vi "Set DBC Communication.vi"(8 "error in":errorcluster, 10 "DBC Communication.lvclass":refnum<class "DBC Communication.lvclass">, 11 "HSU MCU V2 in":refnum<class "HSU MCU V2.lvclass">) -> (0 "error out":errorcluster, 3 "HSU MCU V2 out":refnum<class "HSU MCU V2.lvclass">)   [LabVIEW 2024, in "HSU MCU V2.lvclass"]
uses:
  HSU MCU V2.lvclass
  DBCCommunication/DBC Communication.lvclass
  HSU MCU V2.lvclass/HSU MCU V2.ctl
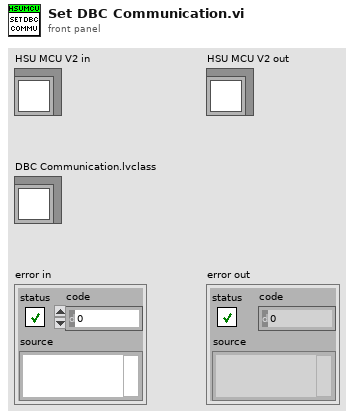
[diagram p1: front panel]
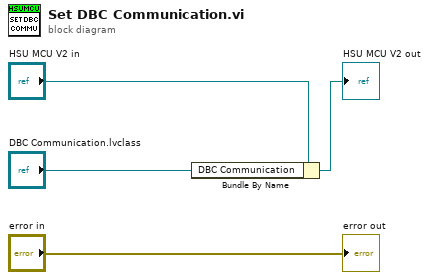
[diagram p0: block diagram]
diagram:
  n1 = Bundle By Name(cluster="HSU MCU V2 in", "DBC Communication"="DBC Communication.lvclass") -> (→"HSU MCU V2 out":refnum<class "HSU MCU V2.lvclass">)
  "error out" <- "error in"
